vi "IP Checksum.vi"(10 "Packet (String)":string, 11 "Packet (U8)":u8[](array[numeric]) format="%02x") -> (0 "Valid Packet?":bool, 1 "Packet+cksum (U8)":u8[](array[numeric]) format="%02x", 2 "cksum (U16)":u16 format="%x", 3 "cksum (U8 Array)":u8[](array[numeric]))   [LabVIEW 2018]
panel:
  out "16 bit 1's complement":u32 format="%04x"
  out "2's complement sum":u32 format="%08x"
  out "16 bit words":u16[](array[numeric]) format="%04x"
  # "IP Checksum.vi - Calculates IP-style checksums on a block of data"
  # "1's complement of the 1's complement sum"
  # "Indicates a valid\nincoming packet\nwas processed"
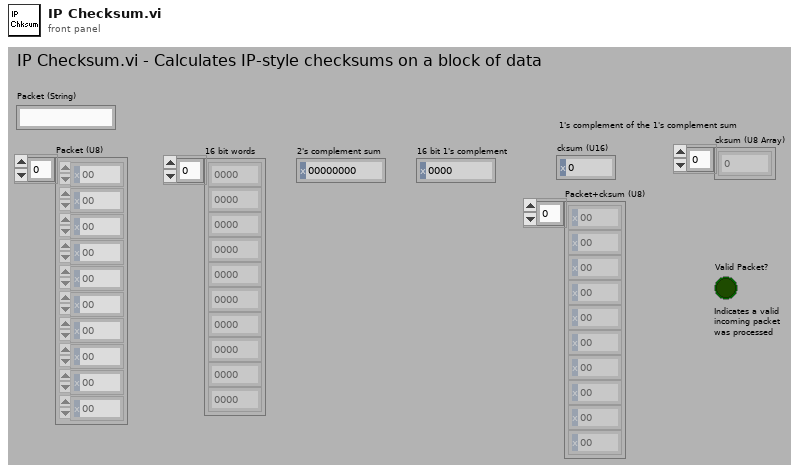
[diagram p1: front panel]
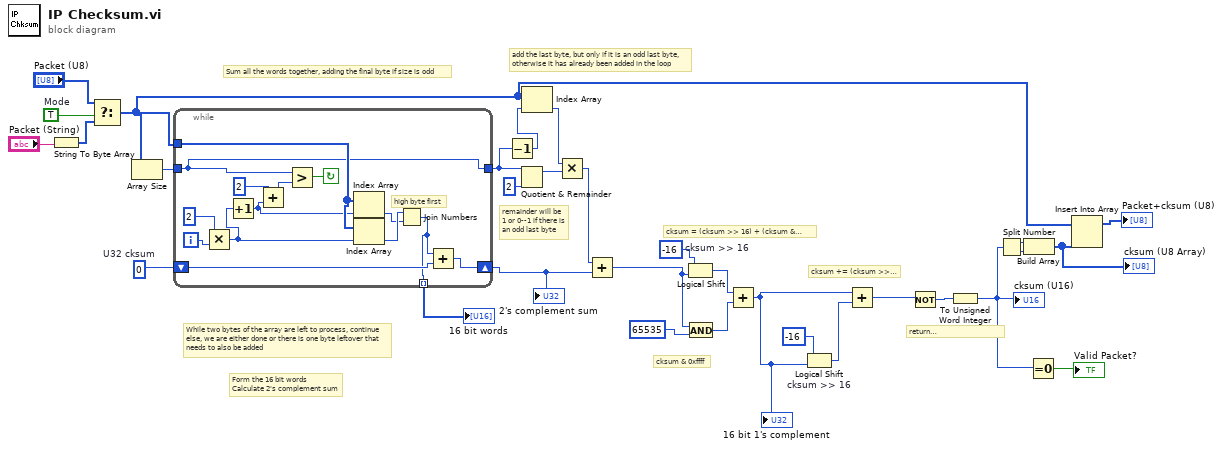
[diagram p0: block diagram]
diagram:
  w13 = TRUE  # Mode
  w24 = u32 0  # U32 cksum
  # "Form the 16 bit words\nCalculate 2's complement sum"
  # "cksum = (cksum >> 16) + (cksum & 0xffff);"
  # "remainder will be\n1 or 0--1 if there is\nan odd last byte"
  # "add the last byte, but only if it is an odd last byte,\notherwise it has already been added in the loop"
  # "Sum all the words together, adding the final byte if size is odd"
  # "While two bytes of the array are left to process, continue\nelse, we are either done or there is one byte leftover that\nneeds to also be added"
  # "return (USHORT)(~cksum);"
  # "cksum += (cksum >> 16);"
  # "cksum & 0xffff"
  n1 = String To Byte Array(string="Packet (String)") -> (unsigned byte array=w15:u8[])
  n2 = Select(t="Packet (U8)", s=w13, f=w15) -> (s? t:f=w6:u8[])
  n3 = Array Size(array=w6) -> (size(s)=w25:i32)
  n4 = while {
    tunnel: w25 -> [w36]
    tunnel: w6 -> [w37]
    shift-right: [w38] -> w20
    shift-left: w24 -> [w39]
    tunnel: [w36] -> w16
    tunnel: [w32] -> w8 mode=indexing
    i -> [w45]
    stop <- w42 continue-if-true
    # "high byte first"
    n5 = Multiply(x=2, y=w45) -> (x*y=w43:i32)
    n6 = Increment(x=w43) -> (x+1=w35:i32)
    n7 = Add(x=2, y=w35) -> (x+y=w34:i32)
    n8 = Greater?(x=w36, y=w34) -> (0:w42:bool)
    n9 = Index Array(array=w37, index=w35) -> (element=w40:u8)
    n10 = Index Array(array=w37, index=w43) -> (element=w41:u8)
    n11 = Join Numbers(hi=w41, lo=w40) -> ((hi.lo)=w32:u16)
    n12 = Add(x=w32, y=w39) -> (x+y=w38:u32)
  }
  "16 bit words" <- w8
  "2's complement sum" <- w20
  n13 = Decrement(x=w16) -> (x-1=w17:i32)
  n14 = Quotient & Remainder(x=w16, y=2) -> (x-y*floor(x/y)=w21:i32)  [unwired: 1 out]
  n15 = Index Array(array=w6, index=w17) -> (element=w22:u8)
  n16 = Multiply(x=w22, y=w21) -> (x*y=w19:i32)
  n17 = Add(x=w19, y=w20) -> (x+y=w12:u32)
  n18 = Logical Shift "cksum >> 16"(y=-16 ("x"), x=w12) -> (x << y=w30:u32)
  n19 = And(x=w12, y=u32 65535) -> (x .and. y?=w29:u32)
  n20 = Add(x=w30, y=w29) -> (x+y=w9:u32)
  "16 bit 1's complement" <- w9
  n21 = Logical Shift "cksum >> 16"(y=-16 ("x"), x=w9) -> (x << y=w28:u32)
  n22 = Add(x=w9, y=w28) -> (x+y=w27:u32)
  n23 = Not(x=w27) -> (.not. x?=w26:u32)
  n24 = To Unsigned Word Integer(number=w26) -> (unsigned 16bit integer=w2:u16)
  "cksum (U16)" <- w2
  n25 = Split Number(x=w2) -> (hi(x)=w4:u8, lo(x)=w5:u8)
  n26 = Build Array(w4, w5) -> (w3:u8[])
  "cksum (U8 Array)" <- w3
  n27 = Equal To 0?(x=w2) -> (x = 0?=→"Valid Packet?":bool)
  n28 = Insert Into Array(array=w6, new element=w3) -> (→"Packet+cksum (U8)":u8[])  [unwired: 1 in]
